vi "ReplaceCommaToDot.vi"() -> ()   [LabVIEW 2019]
panel:
  in  "Path":path
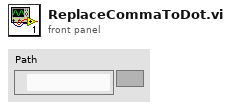
[diagram p1: front panel]
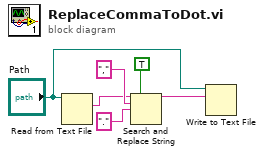
[diagram p0: block diagram]
diagram:
  n1 = Read from Text File(file (use dialog)="Path") -> (text=w1:string)  [unwired: 3 in, 3 out]
  n2 = Search and Replace String(replace all?=TRUE ("replace all? (F)"), input string=w1, search string="," ("format string"), replace string="." ("replace string (\"\")")) -> (result string=w5:string)  [unwired: 4 in, 3 out]
  n3 = Write to Text File(file (use dialog)="Path", text=w5) -> ()  [unwired: 2 in, 3 out]
